vi "IndependentAEcollector.vi"() -> ()   [LabVIEW 2009]
uses:
  <vilib>/Waveform/WDTOps.llb/WDT Waveform to XY Pairs DBL.vi
  <vilib>/express/express analysis/Spectral/XNode/ExpressSpectralMeasurementsBlockNode.xnode
  <vilib>/express/express analysis/Spectral/Block/exnSpectralBlock spectral measurements peak poly.vi
  <vilib>/express/express analysis/Spectral/Block/exnSpectralBlock spectral measurements peak DDT.vi
panel:
  out "Meter":dbl(knob) scale=0.0..1.0
  in  "stop":bool
  in  "Max Noise VPP":dbl
  out "FFT":dynamicdata(graph)
  out "Waveform Graph":dynamicdata(graph)
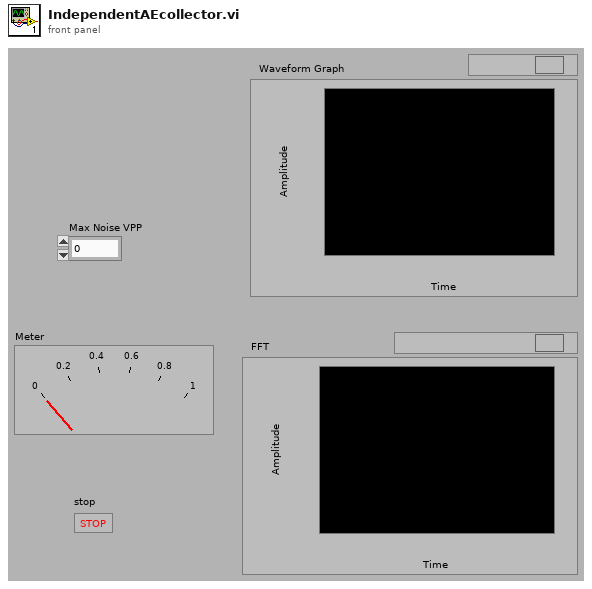
[diagram p1: front panel]
types:
  T1 = enum16{"open", "replace", "create", "open or create", "replace or create", "replace or create with confirmation"}
  T2 = cluster{"averaging mode":u16, "weighting mode":u16, "number of averages":u32}
  T3 = cluster{"dB On (F)":bool, "unwrap phase (F)":bool, "convert to degree (F)":bool}
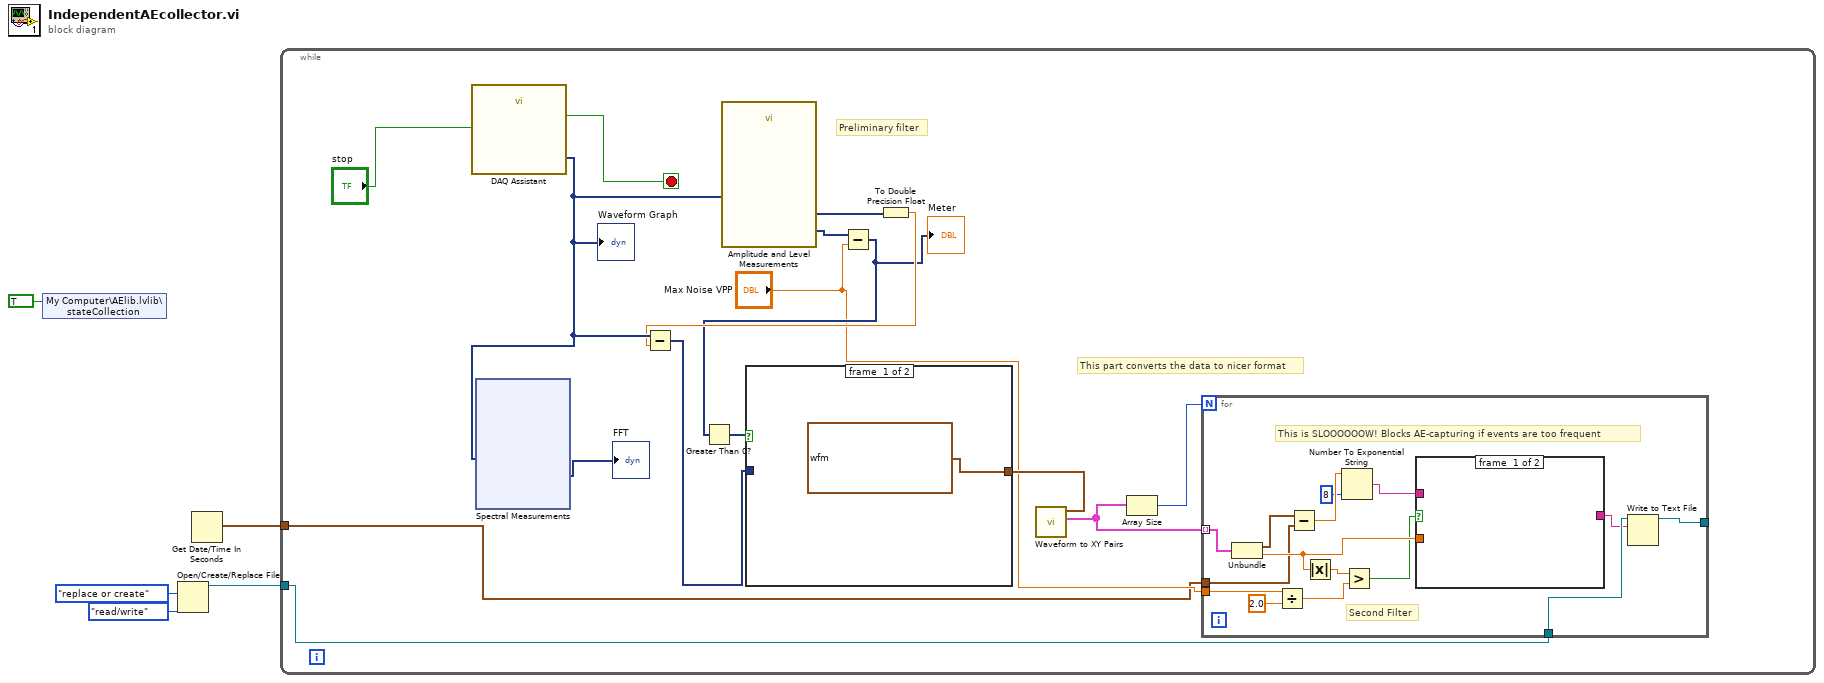
[diagram p0: block diagram]
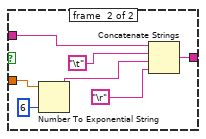
[diagram p2: hidden frame]
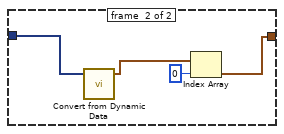
[diagram p3: hidden frame]
diagram:
  n1 = shared-variable "My Computer\\AElib.lvlib\\stateCollection"(TRUE ("stateCollection")) -> ()  [unwired: 1 in, 1 out]
  n2 = Open/Create/Replace File(operation (0:open)=T1."replace or create", access (0:read/write)=enum16{"read/write", "read-only", "write-only"}."read/write") -> (refnum out=w4:refnum<file>)  [unwired: 4 in, 2 out]
  n3 = Get Date/Time In Seconds() -> (seconds since 1Jan1904=w1:timestamp)
  n4 = while {
    tunnel: w4 -> [w8]
    tunnel: w1 -> [w6]
    stop <- w12 stop-if-true
    # "Preliminary filter"
    # "This part converts the data to nicer format"
    n5 = call "DAQ Assistant"("stop (F)"="stop") -> ("data"=w19:dynamicdata, "stopped"=w12:bool)  [unwired: 15 in, 2 out]
    "Waveform Graph" <- w19
    n6 = xnode "Spectral Measurements"("Signals"=w19) -> ("FFT - (Peak)"=→"FFT":dynamicdata)  [unwired: 1 in, 2 out]
    n7 = call "Amplitude and Level Measurements"("Signals"=w19) -> ("Mean (DC)"=w18:dynamicdata, "Peak to Peak"=w15:dynamicdata)  [unwired: 12 in, 1 out]
    n8 = Subtract(x=w15, y="Max Noise VPP") -> (x-y=w14:dynamicdata)
    "Meter" <- w14
    n9 = Greater Than 0?(x=w14) -> (x > 0?=w20:dynamicdata)
    n10 = To Double Precision Float(number=w18) -> (double precision float=w17:dbl)
    n11 = Subtract(x=w19, y=w17) -> (x-y=w13:dynamicdata)
    n12 = case shown="True" w20 {
      tunnel: w13 -> [_ w48]
      tunnel: [waveform(dbl) {"t0"=timestamp(0 s since 1904-01-01), "dt"=1.0, "Y"=[]} ("Waveform") w45] -> w11
      frame #0 {
      }
      frame #1 {
        n13 = call "Convert from Dynamic Data"("Dynamic Data Type"=w48) -> ("Array of Waveform"=w46:waveform(dbl)[])  [unwired: 3 in]
        n14 = Index Array(array=w46, index=0) -> (element=w45:waveform(dbl))
      }
    }
    n15 = call-poly <vilib>:"Waveform to XY Pairs.vi"("waveform in"=w11) -> ("XY pairs"=w9:cluster{"x":timestamp, "y":dbl}[])  [unwired: 8 in, 2 out]
    n16 = Array Size(array=w9) -> (size(s)=w10:i32)
    n17 = for {
      N: w10 -> [_]
      tunnel: w9 -> [w36] mode=indexing
      tunnel: w8 -> [w35]
      tunnel: [w33] -> _
      tunnel: "Max Noise VPP" -> [w30]
      tunnel: w6 -> [w26]
      # "This is SLOOOOOOW! Blocks AE-capturing if events are too frequent"
      # "Second Filter"
      n18 = Unbundle(w36) -> ("x"=w25:timestamp, "y"=w32:dbl)
      n19 = Divide(x=w30, y=2.0) -> (x/y=w29:dbl)
      n20 = Subtract(x=w25, y=w26) -> (x-y=w23:dbl)
      n21 = Absolute Value(x=w32) -> (abs(x)=w31:dbl)
      n22 = Number To Exponential String(number=w23, precision (6)=i16 8) -> (E-format string=w24:string)  [unwired: 2 in]
      n23 = Greater?(x=w31, y=w29) -> (0:w28:bool)
      n24 = case shown="True" w28 {
        tunnel: w32 -> [_ w43]
        tunnel: w24 -> [_ w42]
        tunnel: [_ w39] -> w34
        frame #0 {
        }
        frame #1 {
          n25 = Number To Exponential String(number=w43, precision (6)=i16 6) -> (E-format string=w41:string)  [unwired: 2 in]
          n26 = Concatenate Strings(w42, "\t", w41, "\r") -> (w39:string)
        }
      }
      n27 = Write to Text File(file (use dialog)=w35, text=w34) -> (refnum out=w33:refnum<file>)  [unwired: 2 in, 2 out]
    }
  }
